vi "MoveToNamedPosition.vi"(8 "error in (no error)":errorcluster, 10 "MoveToNamedPosition":T1, 11 "XYStage":refnum<class "XYStage.lvclass">) -> (0 "error out":errorcluster, 3 "XYStage out":refnum<class "XYStage.lvclass">)   [LabVIEW 2013, in "XYStage.lvclass"]
doc: "---------------------------------------------------------------\nJKI State Machine Objects™\nhttp://jki.net/state-machine-objects/\nCopyright (C) 2005-2015, JKI <info@jki.net>\nALL RIGHTS RESERVEDJKI State Machine Objects (SMO) 1.0.0.4\nJKI - JKI\nCopyright (c) 2015, JKI"
uses:
  XYStage.lvclass
  Typedefs/PrivateEvents--XYStage.MoveToNamedPosition.ctl
panel:
  # "For instructions on how to use the JKI State Machine Objects, examples and video tutorials, visit:\nhttp://jki.net/state-machine-objects/\n\nJKI State Machine Objects™\nhttp://jki.net/state-machine-objects/\nCopyright (C) 2005-2015, JKI <info@jki.net>\nALL RIGHTS RESERVED"
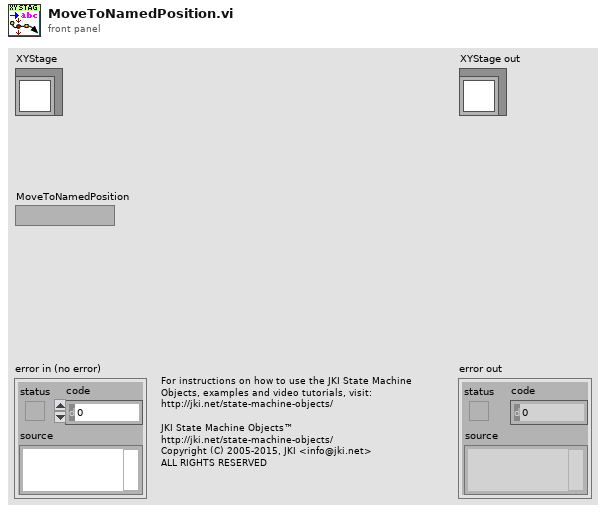
[diagram p1: front panel]
types:
  T1 = typedef "XYStage.lvclass/PrivateEvents--XYStage.MoveToNamedPosition.ctl" = string
  T2 = typedef "XYStage.lvclass/(real)Coords--Cluster.ctl" = cluster{"X":dbl, "Y":dbl}
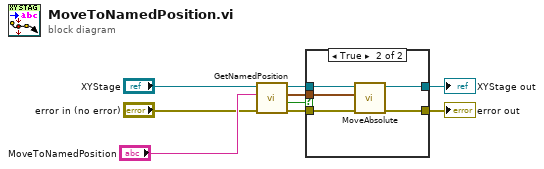
[diagram p0: block diagram]
diagram:
  n1 = call "GetNamedPosition.vi"("error in (no error)"="error in (no error)", "Name"="MoveToNamedPosition", "XYStage"="XYStage") -> ("error out"=w3:errorcluster, "exists"=w1:bool, "Position"=w6:T2, "XYStage out"=w5:refnum<class "XYStage.lvclass">)  [unwired: 5 in]
  n2 = case shown="True" w1 {
    tunnel: w6 -> [_ w16]
    tunnel: w5 -> [w11 w15]
    tunnel: [w11 w14] -> w4
    tunnel: w3 -> [w10 w13]
    tunnel: [w10 w12] -> w2
    frame False {
    }
    frame True {
      n3 = call "MoveAbsolute.vi"("error in (no error)"=w13, "Units"=w16, "XYStage"=w15) -> ("error out"=w12:errorcluster, "XYStage out"=w14:refnum<class "XYStage.lvclass">)  [unwired: 7 in]
    }
  }
  "error out" <- w2
  "XYStage out" <- w4
